vi "Mouse Up - Begin Edit Cell.vi"(8 "error in (no error)":errorcluster, 9 "Valid Region":T1={"left"=-1, "top"=-1, "right"=-1, "bottom"=-1}, 10 "Coords":T2, 11 "MCListbox with Checkboxes in":refnum<class "MCListbox with Checkboxes.lvclass">) -> (0 "error out":errorcluster, 2 "Edit Started?":bool, 3 "MCListbox with Checkboxes out":refnum<class "MCListbox with Checkboxes.lvclass">)   [LabVIEW 2016, in "MCListbox with Checkboxes.lvclass"]
uses:
  MCListbox with Checkboxes.lvclass
  <vilib>/Utility/miscctls.llb/LVPoint32TypeDef.ctl
  MCListbox with Checkboxes.lvclass/MCListbox with Checkboxes.ctl
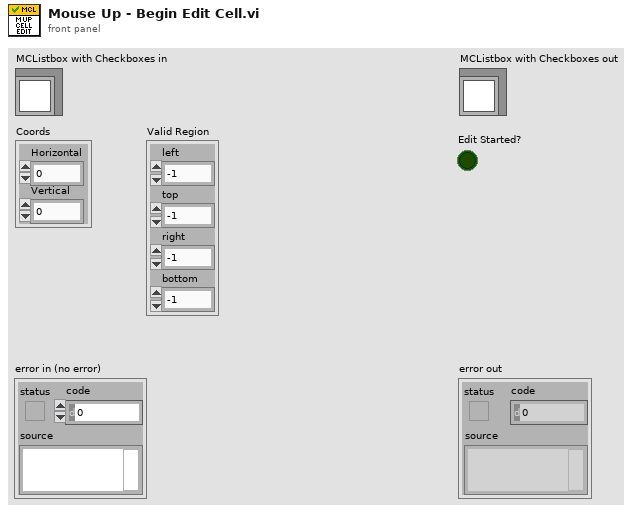
[diagram p1: front panel]
types:
  T1 = cluster{"left":i16, "top":i16, "right":i16, "bottom":i16}
  T2 = typedef "LVPoint32TypeDef.ctl" = cluster{"Horizontal":i32, "Vertical":i32}
  T3 = cluster{"left":bool, "top":bool, "right":bool, "bottom":bool}
  T4 = typedef "LVRowAndColumnTypeDef.ctl" = cluster{"Row":i32, "Column":i32}
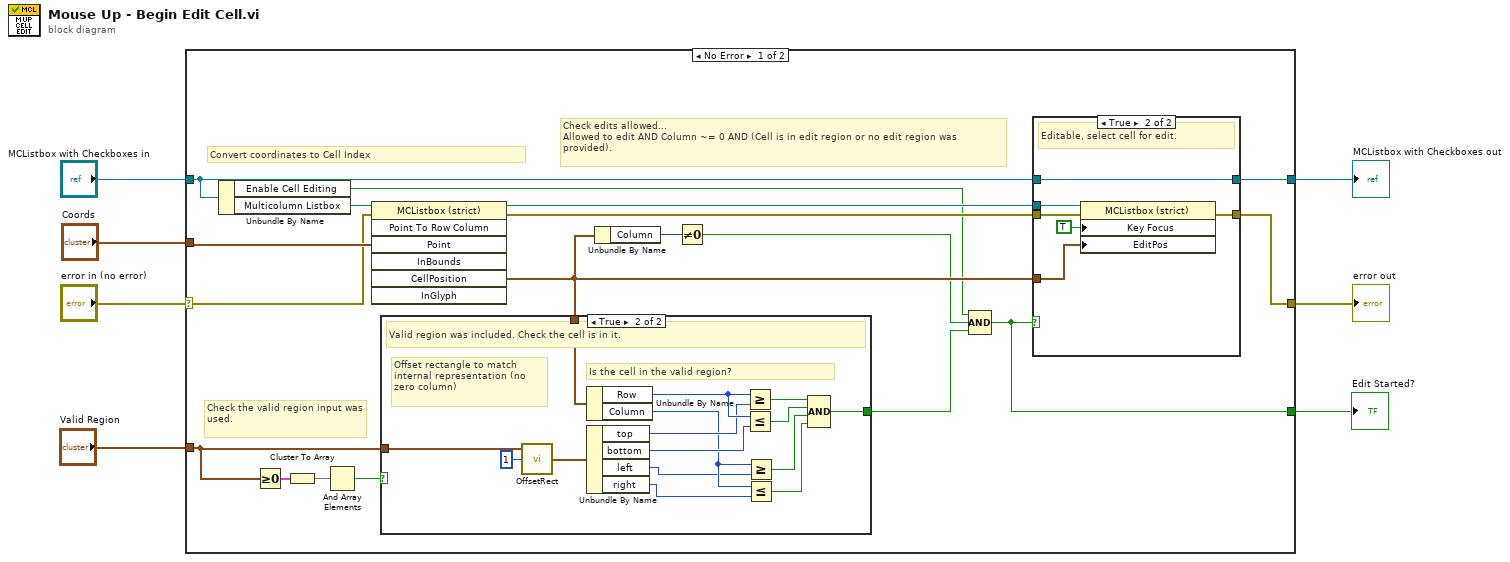
[diagram p0: block diagram]
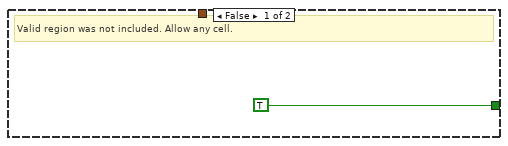
[diagram p2: hidden frame]
diagram:
  n1 = case shown="No Error" "error in (no error)" {
    selector: "error in (no error)" -> [w14 w51]
    tunnel: [w24 w51] -> w6
    tunnel: [w25 w50] -> w5
    tunnel: "MCListbox with Checkboxes in" -> [w21 w50]
    tunnel: "Coords" -> [w22 _]
    tunnel: "Valid Region" -> [w15 _]
    tunnel: [w8 _] -> w1
    frame No Error {
      # "Convert coordinates to Cell Index"
      # "Check edits allowed...\nAllowed to edit AND Column ~= 0 AND (Cell is in edit region or no edit region was provided)."
      # "Check the valid region input was used."
      n2 = Unbundle By Name(w21) -> ("Enable Cell Editing"=w13:bool, "Multicolumn Listbox"=w23:refnum<vi>)
      n3 = Greater Or Equal To 0?(x=w15) -> (x >= 0?=w17:T3)
      n4 = Cluster To Array(cluster=w17) -> (array=w16:bool[])
      n5 = And Array Elements(Boolean array=w16) -> (logical AND=w9:bool)
      n6 = invoke class="MCListbox (strict)" method="Point To Row Column"(reference=w23, error in=w14, "Point"=w22) -> (reference out=w18:refnum<vi>, error out=w20:errorcluster, "CellPosition"=w19:T4)  [unwired: 4 in, 4 out]
      n7 = case shown="True" w9 {
        tunnel: w19 -> [_ w41]
        tunnel: w15 -> [_ w40]
        tunnel: [TRUE w27] -> w10
        frame False {
          # "Valid region was not included. Allow any cell."
        }
        frame True {
          # "Is the cell in the valid region?"
          # "Offset rectangle to match internal representation (no zero column)"
          # "Valid region was included. Check the cell is in it."
          n8 = call <vilib>:"OffsetRect.vi"("h"=i16 1, "rect"=w40) -> ("offset rect"=w38:T1)  [unwired: 1 in]
          n9 = Unbundle By Name(w41) -> ("Row"=w37:i32, "Column"=w34:i32)
          n10 = Unbundle By Name(w38) -> ("top"=w36:i16, "bottom"=w35:i16, "left"=w33:i16, "right"=w32:i16)
          n11 = Greater Or Equal?(x=w37, y=w36) -> (x >= y?=w31:bool)
          n12 = Less Or Equal?(x=w37, y=w35) -> (x <= y?=w30:bool)
          n13 = Greater Or Equal?(x=w34, y=w33) -> (x >= y?=w29:bool)
          n14 = Less Or Equal?(x=w34, y=w32) -> (x <= y?=w28:bool)
          n15 = Compound Arithmetic op=AND(w31, w30, w29, w28) -> (w27:bool)
        }
      }
      n16 = Unbundle By Name(w19) -> ("Column"=w12:i32)
      n17 = Not Equal To 0?(x=w12) -> (x != 0?=w11:bool)
      n18 = Compound Arithmetic op=AND(w13, w11, w10) -> (w8:bool)
      n19 = case shown="True" w8 {
        tunnel: w21 -> [w43 w49]
        tunnel: [w43 w49] -> w25
        tunnel: w20 -> [w42 w48]
        tunnel: [w42 w46] -> w24
        tunnel: w18 -> [_ w47]
        tunnel: w19 -> [_ w45]
        frame False {
          # "Not editable, do nothing."
        }
        frame True {
          # "Editable, select cell for edit."
          n20 = property class="MCListbox (strict)"(reference=w47, error in=w48, "Key Focus"=TRUE, "EditPos"=w45) -> (error out=w46:errorcluster)  [unwired: 1 out]
        }
      }
    }
    frame Error {
    }
  }
  "error out" <- w6
  "MCListbox with Checkboxes out" <- w5
  "Edit Started?" <- w1
